vi "Variant Cluster to Array.vi"(8 "error in (no error)":errorcluster, 11 "Cluster":variant) -> (0 "error out":errorcluster, 3 "Array":variant[](array[variant]))   [LabVIEW 2020, in "DSF Configuration Utility.lvlib"]
uses:
  DSF Configuration Utility.lvlib
  <vilib>/Utility/Data Type/NI_Data Type.lvlib
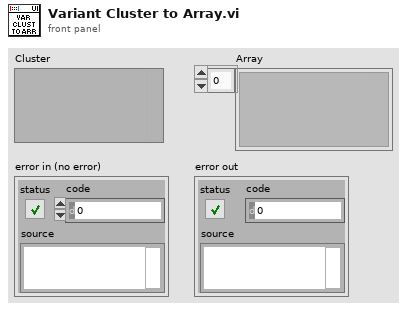
[diagram p1: front panel]
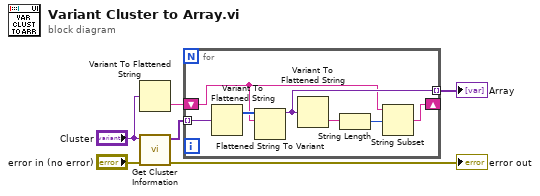
[diagram p0: block diagram]
diagram:
  n1 = Variant To Flattened String(Variant="Cluster") -> (data string=w1:string)  [unwired: 1 out]
  n2 = call <vilib>:"Get Cluster Information.vi"("error in (no error)"="error in (no error)", "variant"="Cluster") -> ("error out"=→"error out":errorcluster, "cluster elements"=w4:variant[])  [unwired: 8 in]
  n3 = for {
    tunnel: w4 -> [w13] mode=indexing
    tunnel: [w11] -> w2 mode=indexing
    shift-right: [w7] -> _
    shift-left: w1 -> [w10]
    n4 = Variant To Flattened String(Variant=w13) -> (1:w12:i16[])  [unwired: 1 out]
    n5 = Flattened String To Variant(6:w10, 7:w12) -> (3:w11:variant)  [unwired: 1 in, 1 out]
    n6 = Variant To Flattened String(Variant=w11) -> (data string=w9:string)  [unwired: 1 out]
    n7 = String Length(string=w9) -> (length=w8:i32)
    n8 = String Subset(string=w10, offset (0)=w8) -> (substring=w7:string)  [unwired: 1 in]
  }
  "Array" <- w2
